vi "derivative.vi"(9 "temperature (min)":dbl[](array[numeric])=[1.0, 2.0, 3.0, 4.0, 5.0, 6.0, 7.0, 8.0, 9.0, 10.0], 10 "frequency (kHz)":dbl[](array[numeric])=[1.0, 2.0, 3.0, 3.0, 4.0, 5.0, 5.0, 6.0, 7.0, 8.0]) -> (3 "derivative (kHz/min)":dbl[](array[numeric])=[0.0, 1.0, 1.0, 0.0, 1.0, 1.0, 0.0, 1.0, 1.0, 1.0])   [LabVIEW 2015]
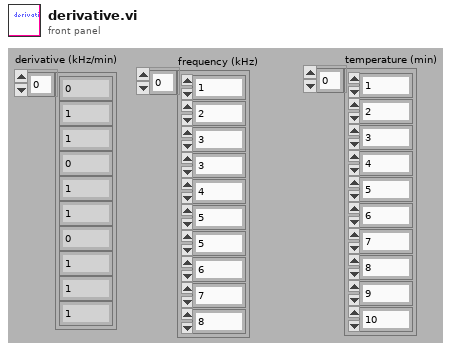
[diagram p1: front panel]
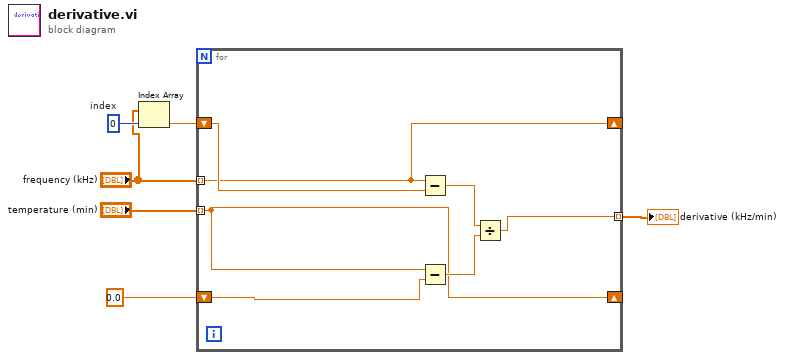
[diagram p0: block diagram]
diagram:
  w6 = 0  # index
  n1 = Index Array(array="frequency (kHz)", index=w6) -> (element=w5:dbl)
  n2 = for {
    shift-right: [w12] -> _
    shift-left: w5 -> [w13]
    shift-right: [w7] -> _
    shift-left: 0.0 -> [w11]
    tunnel: "frequency (kHz)" -> [w12] mode=indexing
    tunnel: "temperature (min)" -> [w7] mode=indexing
    tunnel: [w8] -> w1 mode=indexing
    n3 = Subtract(x=w12, y=w13) -> (x-y=w10:dbl)
    n4 = Subtract(x=w7, y=w11) -> (x-y=w9:dbl)
    n5 = Divide(x=w10, y=w9) -> (x/y=w8:dbl)
  }
  "derivative (kHz/min)" <- w1
